vi "Configure Math (Dual).vi"(7 "Operator (0: ADD)":u16(ring) items=["ADD", "SUBTRACT", "MULTIPLY", "DIVIDE"], 8 "error in (no error)":errorcluster, 9 "2nd Source (1: Channel 2)":u16(ring)=1 items=["Channel 1"=0, "Channel 2"=1, "Channel 3"=2, "Channel 4"=3, "Reference 1"=5, "Reference 2"=6, "Reference 3"=7, "Reference 4"=8], 10 "1st Source (0: Channel 1)":u16(ring) items=["Channel 1"=0, "Channel 2"=1, "Channel 3"=2, "Channel 4"=3, "Reference 1"=5, "Reference 2"=6, "Reference 3"=7, "Reference 4"=8], 11 "VISA resource name":refnum<visa-resource-name>) -> (0 "error out":errorcluster, 3 "VISA resource name out":refnum<visa-resource-name>)   [LabVIEW 2016, in "Tektronix DPO MSO 2000 4000 Series.lvlib"]
doc: "Configures a math channel for standard waveform math operations."
uses:
  Tektronix DPO MSO 2000 4000 Series.lvlib
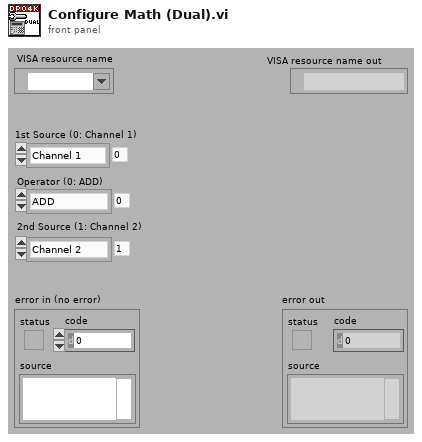
[diagram p1: front panel]
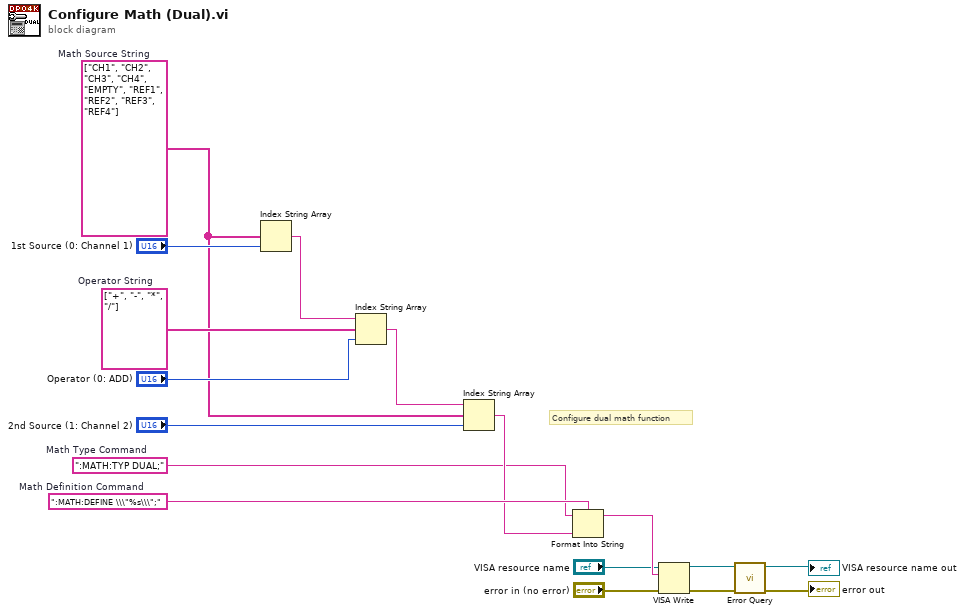
[diagram p0: block diagram]
diagram:
  w3 = string[] ["CH1", "CH2", "CH3", "CH4", "EMPTY", "REF1", "REF2", "REF3", "REF4"]  # Math Source String
  w7 = ":MATH:TYP DUAL;"  # Math Type Command
  w13 = ":MATH:DEFINE \\\"%s\\\";"  # Math Definition Command
  w15 = string[] ["+", "-", "*", "/"]  # Operator String
  # "Configure dual math function"
  n1 = Index String Array(1:"1st Source (0: Channel 1)", 2:w3) -> (0:w4:string)  [unwired: 1 in]
  n2 = Index String Array(1:"Operator (0: ADD)", 2:w15, 3:w4) -> (0:w14:string)
  n3 = Index String Array(1:"2nd Source (1: Channel 2)", 2:w3, 3:w14) -> (0:w12:string)
  n4 = Format Into String(format string=w13, initial string=w7, w12) -> (resulting string=w6:string)  [unwired: 1 in, 1 out]
  n5 = VISA Write(VISA resource name="VISA resource name", write buffer=w6, error in (no error)="error in (no error)") -> (VISA resource name out=w11:refnum<visa-resource-name>, error out=w10:errorcluster)  [unwired: 1 out]
  n6 = call "Error Query.vi"("error in (no error)"=w10, "VISA resource name"=w11) -> ("error out"=→"error out":errorcluster, "VISA resource name out"=→"VISA resource name out":refnum<visa-resource-name>)  [unwired: 6 in, 2 out]
